vi "Untitled 1.vi"() -> ()   [LabVIEW 2011]
panel:
  out "appended array":dbl[](array[numeric])
  in  "Paso":dbl
  in  "Tiempo":dbl
  in  "Kp2":dbl
  in  "Kp1":dbl
  in  "Zigmae":dbl[](array[numeric])
  in  "Q":dbl
  in  "Vr/Wr":dbl[](array[numeric])
  out "PhiL":dbl
  out "PhiR":dbl
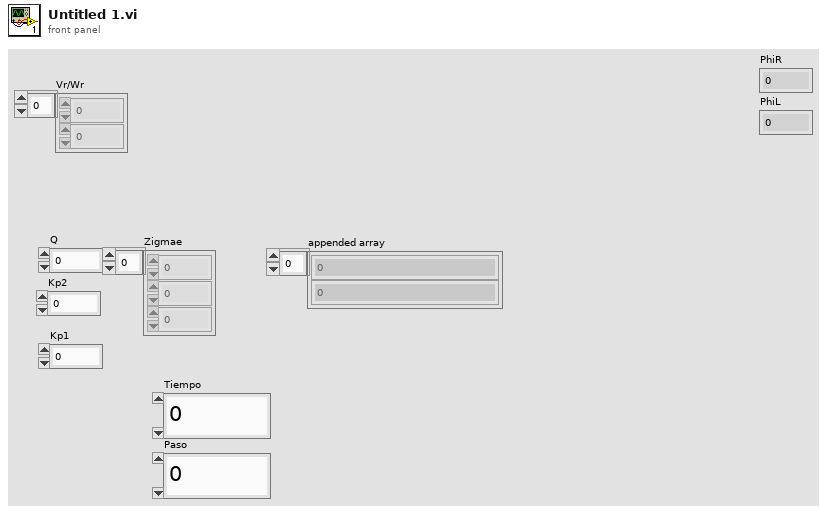
[diagram p1: front panel]
types:
  T1 = typedef "NI_Matrix.lvlib/RealMatrix.ctl" = dbl[][]
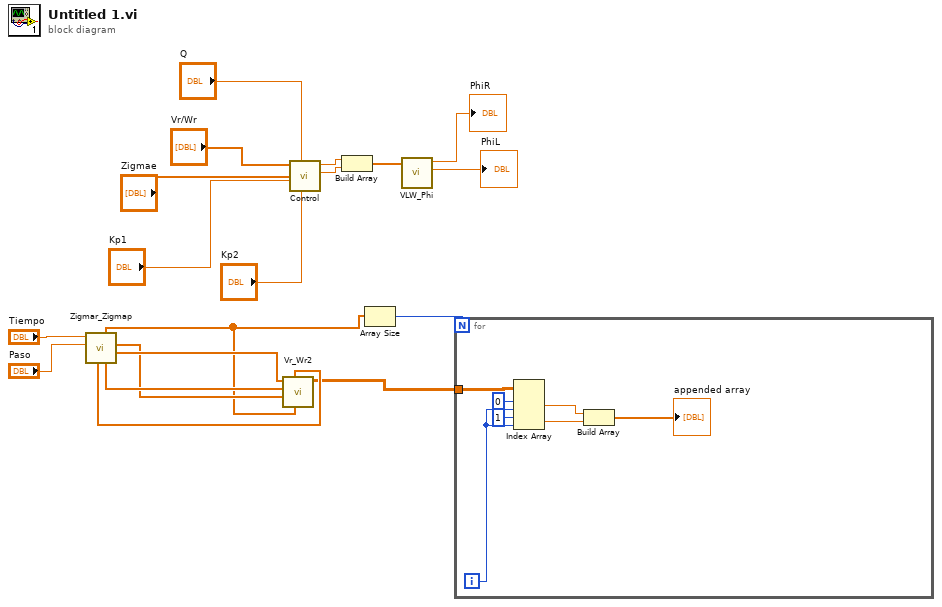
[diagram p0: block diagram]
diagram:
  n1 = call "Zigmar_Zigmap.vi"("Paso"="Paso", "Tiempo"="Tiempo") -> ("Xdrp"=w7:dbl[], "Phir"=w5:dbl[], "Ydrp"=w6:dbl[], "Xdr"=w2:dbl[], "Phirp"=w4:dbl[])  [unwired: 4 in, 1 out]
  n2 = call "Vr_Wr2.vi"("Xdr"=w2, "Phirp"=w4, "Phir"=w5, "Ydrp"=w6, "Xdrp"=w7) -> ("Real Matrix"=w1:T1)  [unwired: 6 in]
  n3 = call "Control.vi"("Kp2"="Kp2", "Q"="Q", "Kp1"="Kp1", "Zigmae"="Zigmae", "Vr/Wr"="Vr/Wr") -> ("W"=w17:dbl, "V"=w18:dbl)  [unwired: 5 in]
  n4 = Build Array(w18, w17) -> (w19:dbl[])
  n5 = Array Size(array=w2) -> (size(s)=w3:i32)
  n6 = call "VLW_Phi.vi"("VL/W"=w19) -> ("PhiL"=→"PhiL":dbl, "PhiR"=→"PhiR":dbl)  [unwired: 9 in]
  n7 = for {
    N: w3 -> [_]
    tunnel: w1 -> [w26]
    i -> [w25]
    n8 = Index Array(array=w26, index (row) #1=0 ("index (row)"), index (col) #1=w25, index (row) #2=1 ("index (row)"), index (col) #2=w25) -> (element #1=w22:dbl, element #2=w21:dbl)
    n9 = Build Array(w22, w21) -> (→"appended array":dbl[])
  }
